vi "Global CORR.vi"() -> ()   [LabVIEW 2019]
panel:
  in  "coeff correz":T1={"H1 (QH)"=1.0, "H2 (QH)"=1.0, "H1 (NPSH)"=1.0, "H2 (NPSH)"=1.0, "Abilita\\disabilita"=FALSE}
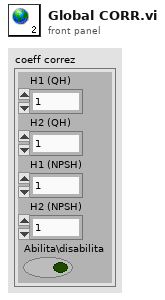
[diagram p1: front panel]
types:
  T1 = cluster{"H1 (QH)":dbl, "H2 (QH)":dbl, "H1 (NPSH)":dbl, "H2 (NPSH)":dbl, "Abilita\\disabilita":bool}
diagram:
